vi "solar_app Launch VI.vi"(4 "Control Values":variant[](array[variant]), 5 "Run Options":T1={"Wait Until Done? (F)"=FALSE, "Auto Dispose Ref? (T)"=TRUE}, 6 "Control Names":string[](array[string]), 7 "Static VI Refnum":refnum<vi>, 8 "error in (no error)":errorcluster, 9 "Open FP? (Ignore)":enum8{"Ignore", "Before", "After"}(ring), 10 "Reentrant Execution? (F)":bool, 11 "VI Name":string) -> (0 "error out":errorcluster, 3 "VI Refnum out":refnum<vi>)   [LabVIEW 2018]
doc: "This VI launches a VI."
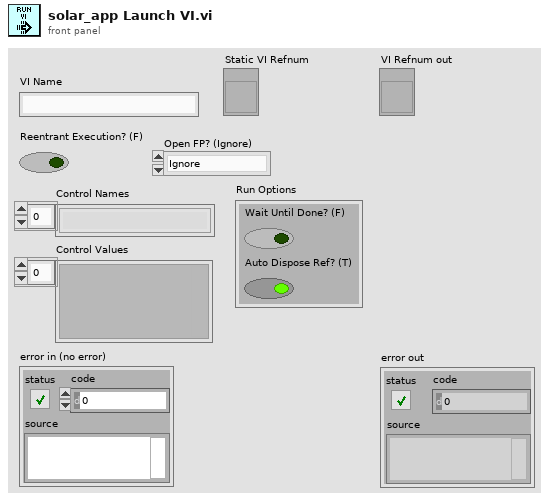
[diagram p1: front panel]
types:
  T1 = cluster{"Wait Until Done? (F)":bool, "Auto Dispose Ref? (T)":bool}
  T2 = enum32{"Bad", "Idle", "Run top level", "Running"}
  T3 = enum32{"Invalid", "Standard", "Closed", "Hidden", "Minimized", "Maximized"}
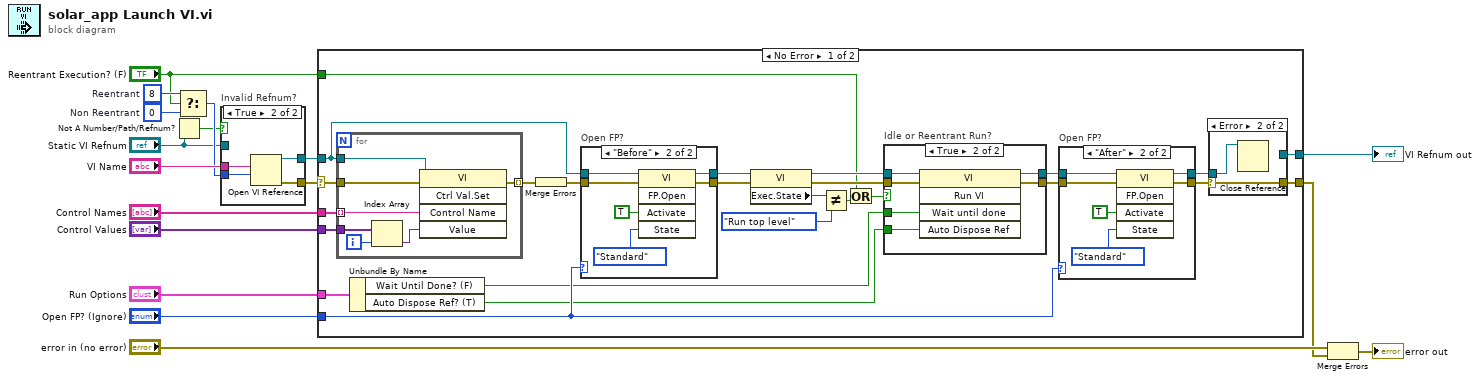
[diagram p0: block diagram]
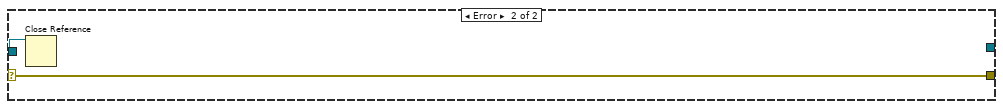
[diagram p7: hidden frame]
diagram:
  w14 = 8  # Reentrant
  w15 = 0  # Non Reentrant
  n1 = Not A Number/Path/Refnum?(number/path/refnum="Static VI Refnum") -> (NaN/Path/Refnum?=w6:bool)
  n2 = Select(t=w14, s="Reentrant Execution? (F)", f=w15) -> (s? t:f=w13:i32)
  n3 = case "Invalid Refnum?" shown="True" w6 {
    tunnel: "VI Name" -> [_ w22]
    tunnel: [_ w21] -> w16
    tunnel: w13 -> [_ w20]
    tunnel: [w18 w19] -> w9
    tunnel: "Static VI Refnum" -> [w18 _]
    frame False {
    }
    frame True {
      n4 = Open VI Reference(vi path=w22, options=w20) -> (vi reference=w19:refnum<vi>, error out=w21:errorcluster)  [unwired: 4 in]
    }
  }
  n5 = case shown="No Error" w16 {
    selector: w16 -> [w43 w84]
    tunnel: "Control Names" -> [w42 _]
    tunnel: "Control Values" -> [w41 _]
    tunnel: "Reentrant Execution? (F)" -> [w37 _]
    tunnel: w9 -> [w28 w83]
    tunnel: [w36 w84] -> w2
    tunnel: "Open FP? (Ignore)" -> [w26 _]
    tunnel: [w31 _] -> w7
    tunnel: "Run Options" -> [w25 _]
    frame No Error {
      n6 = for {
        tunnel: [w70] -> w44 mode=indexing
        tunnel: w43 -> [w69]
        tunnel: w28 -> [w68]
        tunnel: w42 -> [w67] mode=indexing
        tunnel: w41 -> [w66]
        i -> [w64]
        n7 = Index Array(array=w66, index=w64) -> (element=w65:variant)
        n8 = invoke class="VI" method="Ctrl Val.Set"(reference=w68, error in=w69, "Control Name"=w67, "Value"=w65) -> (error out=w70:errorcluster)  [unwired: 1 in, 4 out]
      }
      n9 = Unbundle By Name(w25) -> ("Wait Until Done? (F)"=w24:bool, "Auto Dispose Ref? (T)"=w23:bool)
      n10 = Merge Errors(w44) -> (w30:errorcluster)
      n11 = case "Open FP?" shown="\"Before\"" w26 {
        tunnel: [w49 w53] -> w29
        tunnel: [w48 w52] -> w27
        tunnel: w28 -> [w48 w51]
        tunnel: w30 -> [w49 w50]
        frame Default {
        }
        frame "Before" {
          n12 = invoke class="VI" method="FP.Open"(reference=w51, error in=w50, "Activate"=TRUE ("Activate?"), "State"=T3."Standard") -> (reference out=w52:refnum<vi>, error out=w53:errorcluster)  [unwired: 1 in, 3 out]
        }
      }
      n13 = property class="VI"(reference=w27, error in=w29) -> (reference out=w46:refnum<vi>, error out=w47:errorcluster, "Exec.State"=w45:T2)
      n14 = Not Equal?(x=w45, y=T2."Run top level" ("Execution:State")) -> (x != y?=w40:bool)
      n15 = Or(x=w37, y=w40) -> (x .or. y?=w38:bool)
      n16 = case "Idle or Reentrant Run?" shown="True" w38 {
        tunnel: [w71 w75] -> w35
        tunnel: [w72 w76] -> w34
        tunnel: w47 -> [w71 w78]
        tunnel: w46 -> [w72 w77]
        tunnel: w24 -> [_ w74]
        tunnel: w23 -> [_ w73]
        frame False {
        }
        frame True {
          n17 = invoke class="VI" method="Run VI"(reference=w77, error in=w78, "Wait until done"=w74, "Auto Dispose Ref"=w73) -> (reference out=w76:refnum<vi>, error out=w75:errorcluster)  [unwired: 1 in, 3 out]
        }
      }
      n18 = case "Open FP?" shown="\"After\"" w26 {
        tunnel: [w57 w61] -> w33
        tunnel: [w56 w60] -> w32
        tunnel: w34 -> [w56 w59]
        tunnel: w35 -> [w57 w58]
        frame Default {
        }
        frame "After" {
          n19 = invoke class="VI" method="FP.Open"(reference=w59, error in=w58, "Activate"=TRUE ("Activate?"), "State"=T3."Standard") -> (reference out=w60:refnum<vi>, error out=w61:errorcluster)  [unwired: 1 in, 3 out]
        }
      }
      n20 = case shown="Error" w33 {
        selector: w33 -> [w80 w81]
        tunnel: w32 -> [w79 w82]
        tunnel: [w80 w81] -> w36
        tunnel: [w79 _] -> w31
        frame No Error {
        }
        frame Error {
          n21 = Close Reference(reference=w82) -> ()  [unwired: 1 in, 1 out]
        }
      }
    }
    frame Error {
      n22 = Close Reference(reference=w83) -> ()  [unwired: 1 in, 1 out]
    }
  }
  "VI Refnum out" <- w7
  n23 = Merge Errors("error in (no error)", w2) -> (→"error out":errorcluster)
